vi "3.1-Act Client.vi"() -> ()   [LabVIEW 2010]
uses:
  4-High Neurons/4.1-Act Control Typedef.ctl
  4-High Neurons/4.1.0-Datatype Typedef.ctl
  4-High Neurons/4.1.1-Act Joystick.ctl
  4-High Neurons/4.1.2-Act Neuron TD.ctl
  3.0-Global.vi
panel:
  out "error out":errorcluster
  in  "stop":bool
  in  "error in":errorcluster
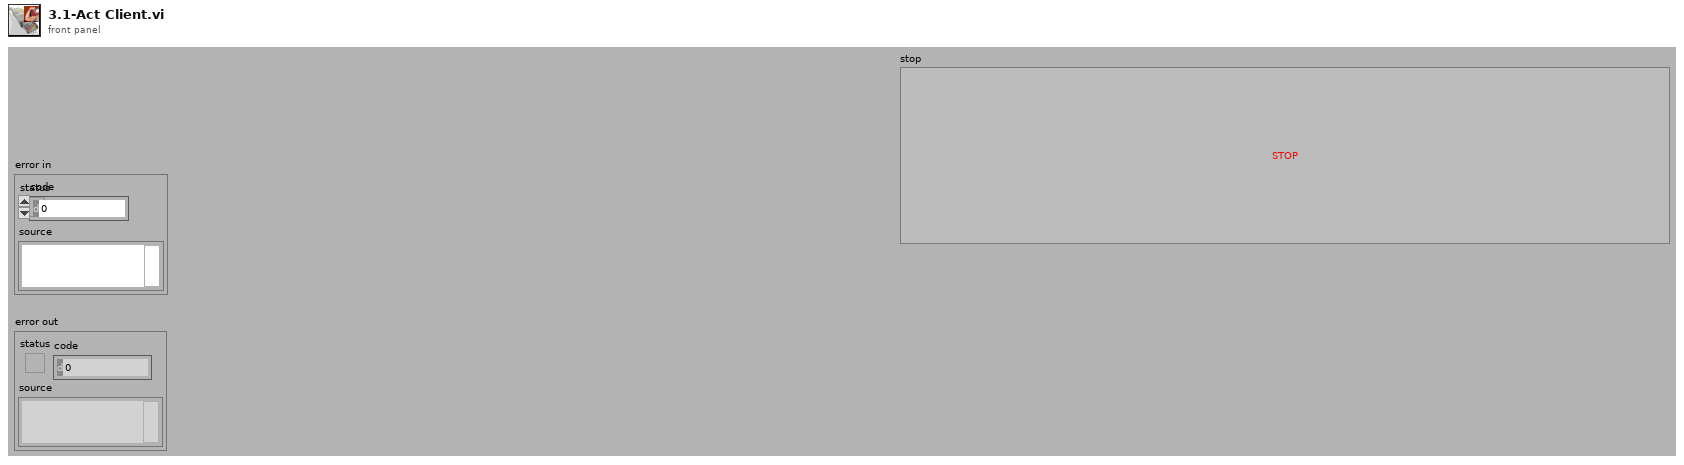
[diagram p1: front panel]
types:
  T1 = typedef "4.1.1-Act Joystick.ctl" = cluster{"Trig":bool, "2":bool, "3":bool, "4":bool, "5":bool, "6":bool, "7":bool, "8":bool, "9":bool, "10":bool, "11":bool, "Pitch":i32, "Ang":bool[], "Wheel":dbl, "Roll":i32, "Yaw":i32, "Left":i32, "Right":i32}
  T2 = typedef "4.1.2-Act Neuron TD.ctl" = cluster{"Speed By Path":dbl[]}
  T3 = typedef "4.1-Act Control Typedef.ctl" = cluster{"4.1.0 Data":variant, "Type of Data":T4, "E-Stop":bool, "Restart":bool, "New IP":bool, "Begin":bool, "Time":i32, "Shutdown":bool}
  T4 = typedef "4.1.0-Datatype Typedef.ctl" = enum16{"4.1.0-Empty Data", "4.1.1-Joystick Data", "4.1.2-Behavioral Data"}
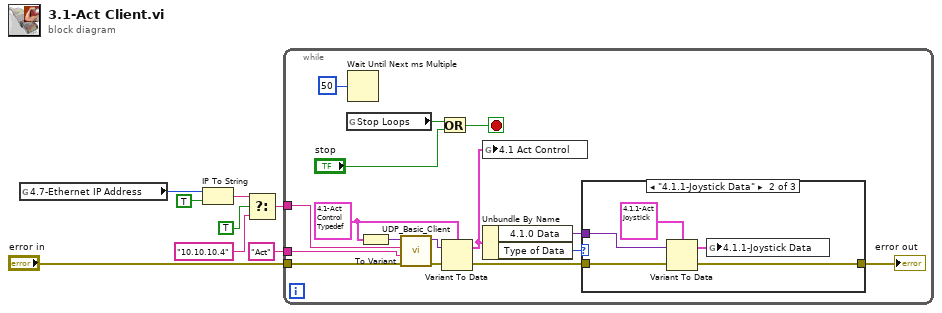
[diagram p0: block diagram]
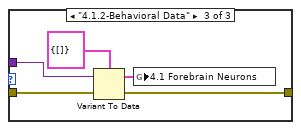
[diagram p3: hidden frame]
diagram:
  n1 = global read "3.0-Global.vi" "4.7-Ethernet IP Address"() -> (w4:u32)
  n2 = IP To String(1:TRUE ("dot notation? (F)"), 2:w4) -> (0:w3:string)
  n3 = Select(t=w3, s=TRUE, f="10.10.10.4") -> (s? t:f=w6:string)
  n4 = while {
    tunnel: "Act" -> [w19]
    tunnel: "error in" -> [w18]
    tunnel: w6 -> [w20]
    stop <- w23 stop-if-true
    w14 = T3 {"4.1.0 Data"=variant, "Type of Data"=enum."4.1.1-Joystick Data", "E-Stop"=FALSE, "Restart"=FALSE, "New IP"=FALSE, "Begin"=FALSE, "Time"=0, "Shutdown"=FALSE} ("4.1 Act Control")
    n5 = global read "3.0-Global.vi" "Stop Loops"() -> (w21:bool)
    n6 = Wait Until Next ms Multiple(millisecond multiple=u32 50) -> ()  [unwired: 1 out]
    n7 = To Variant(anything=w14) -> (Variant=w17:variant)
    n8 = call "UDP_Basic_Client.vi"("error In"=w18, "Service Name"=w19, "IP Adress"=w20, "DataTypeIn"=w17) -> ("error IO"=w15:errorcluster, "DataOut"=w16:variant)  [unwired: 1 in, 1 out]
    n9 = Or(x=w21, y="stop") -> (x .or. y?=w23:bool)
    n10 = Variant To Data(error in=w15, Variant=w16, type=w14) -> (error out=w10:errorcluster, data=w13:T3)
    n11 = global write "3.0-Global.vi" "4.1 Act Control"(w13) -> ()
    n12 = Unbundle By Name(w13) -> ("4.1.0 Data"=w12:variant, "Type of Data"=w11:T4)
    n13 = case shown="\"4.1.1-Joystick Data\"" w11 {
      tunnel: w12 -> [_ w28 w31]
      tunnel: w10 -> [w25 w27 w33]
      tunnel: [w25 w26 w32] -> w9
      frame "4.1.0-Empty Data", Default {
      }
      frame "4.1.1-Joystick Data" {
        n14 = Variant To Data(error in=w27, Variant=w28, type=T1 {"Trig"=FALSE, "2"=FALSE, "3"=FALSE, "4"=FALSE, "5"=FALSE, "6"=FALSE, "7"=FALSE, "8"=FALSE, "9"=FALSE, "10"=FALSE, "11"=FALSE, "Pitch"=0, "Ang"=[], "Wheel"=0.0, "Roll"=0, "Yaw"=0, "Left"=0, "Right"=0} ("Saitek Controler")) -> (error out=w26:errorcluster, data=w29:T1)
        n15 = global write "3.0-Global.vi" "4.1.1-Joystick Data"(w29) -> ()
      }
      frame "4.1.2-Behavioral Data" {
        n16 = Variant To Data(error in=w33, Variant=w31, type=T2 {"Speed By Path"=[]} ("Forebrain Act Neurons")) -> (error out=w32:errorcluster, data=w34:T2)
        n17 = global write "3.0-Global.vi" "4.1 Forebrain Neurons"(w34) -> ()
      }
    }
    "error out" <- w9
  }
